vi "round (Sub VI).vi"(10 "Numeric":dbl, 11 "Number to round":dbl=1234.56789 format="%_9f") -> (3 "Rounded number":dbl=1235.0 format="%_9f")   [LabVIEW 2016]
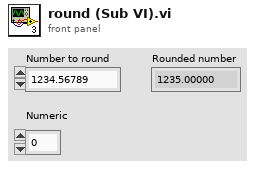
[diagram p1: front panel]
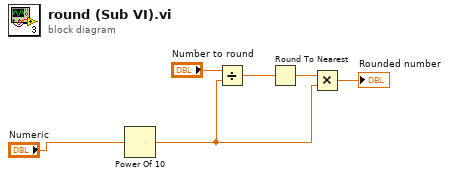
[diagram p0: block diagram]
diagram:
  n1 = Power Of 10(x="Numeric") -> (10^x=w5:dbl)
  n2 = Divide(x="Number to round", y=w5) -> (x/y=w2:dbl)
  n3 = Round To Nearest(number=w2) -> (nearest integer value=w3:dbl)
  n4 = Multiply(x=w3, y=w5) -> (x*y=→"Rounded number":dbl)
